vi "Shutdown_PS1.vi"(3 "error in":errorcluster) -> (7 "Application Dir":path, 8 "COM Port":string, 10 "error out":errorcluster)   [LabVIEW 2015]
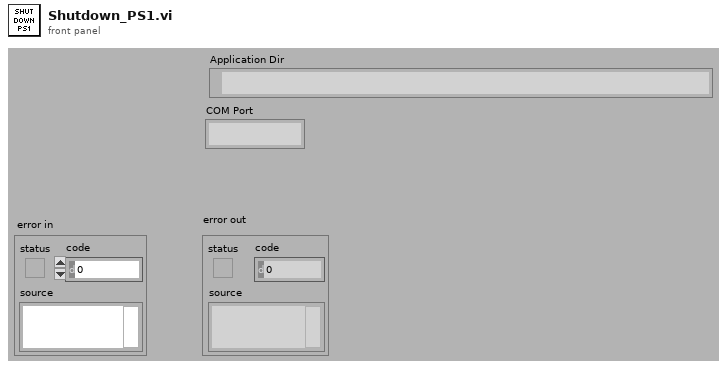
[diagram p1: front panel]
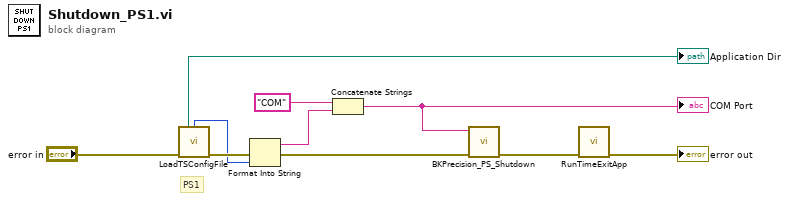
[diagram p0: block diagram]
diagram:
  # "PS1"
  n1 = call "LoadTSConfigFile.vi"("error in (no error)"="error in") -> ("appended path"=→"Application Dir":path, "PS1_COMPort"=w7:i32, "error out"=w10:errorcluster)  [unwired: 4 in, 8 out]
  n2 = Format Into String(error in=w10, w7) -> (resulting string=w8:string, error out=w5:errorcluster)  [unwired: 2 in]
  n3 = Concatenate Strings("COM" ("string"), w8) -> (w6:string)
  "COM Port" <- w6
  n4 = call "BKPrecision_PS_Shutdown.vi"("error in (no error)"=w5, "VISA resource name"=w6) -> ("error out"=w4:errorcluster)  [unwired: 8 in, 1 out]
  n5 = call "RunTimeExitApp.vi"("error in (no error)"=w4) -> ("error out"=→"error out":errorcluster)  [unwired: 10 in]
